vi "create checkpoint file name.vi"(8 "error in (no error)":errorcluster, 10 "name or relative path":string, 11 "Autofocus in":refnum<class "Autofocus.lvclass">) -> (0 "error out":errorcluster, 1 "checkpoint file name":path, 3 "Autofocus out":refnum<class "Autofocus.lvclass">)   [LabVIEW 2012, in "Autofocus.lvclass"]
uses:
  Autofocus.lvclass
  Autofocus.lvclass/Autofocus.ctl
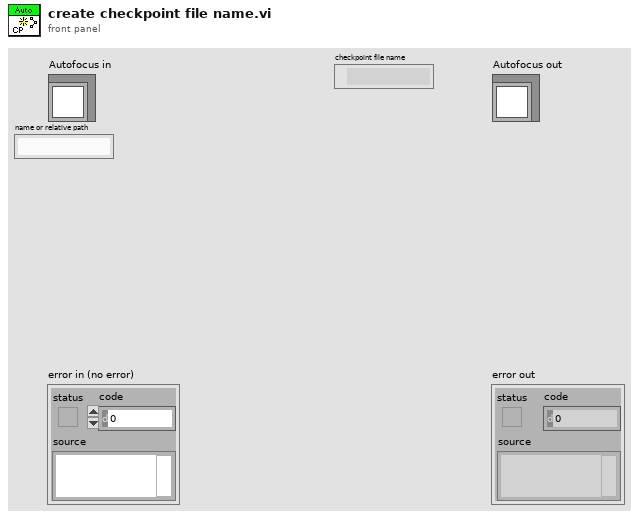
[diagram p1: front panel]
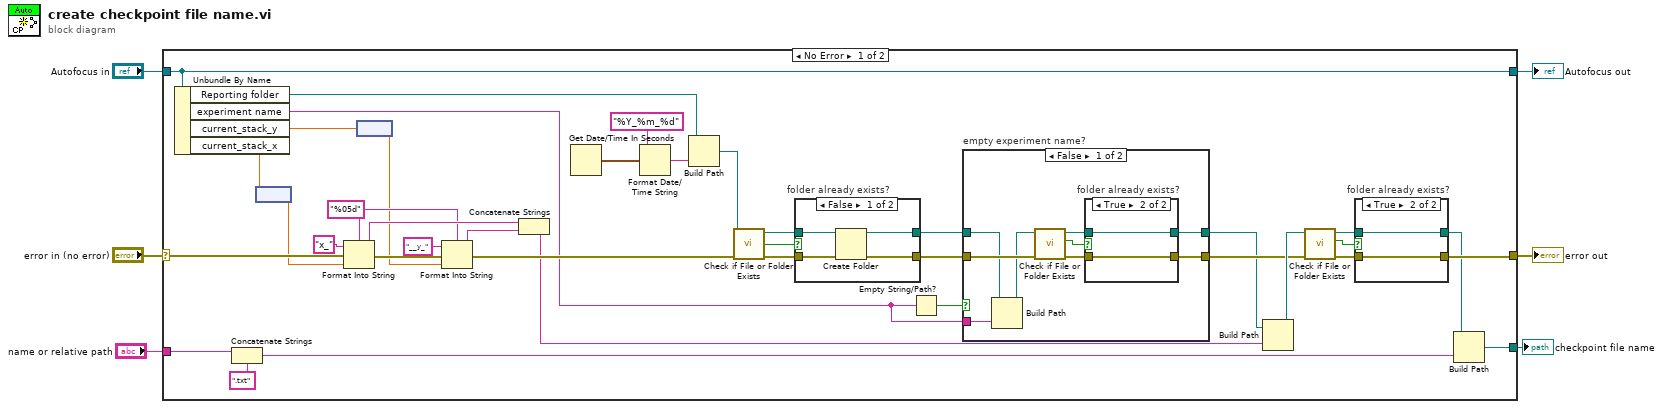
[diagram p0: block diagram]
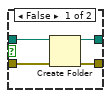
[diagram p2: hidden frame]
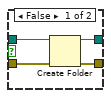
[diagram p4: hidden frame]
diagram:
  n1 = case shown="No Error" "error in (no error)" {
    selector: "error in (no error)" -> [w35 w75]
    tunnel: [w23 w75] -> w5
    tunnel: [w44 w74] -> w3
    tunnel: "Autofocus in" -> [w44 w74]
    tunnel: [w24 _] -> w2
    tunnel: "name or relative path" -> [w21 _]
    frame No Error {
      w41 = "%05d" ("format string")
      n2 = Unbundle By Name(w44) -> ("Reporting folder"=w31:path, "experiment name"=w8:string, "current_stack_y"=w36:dbl[unit], "current_stack_x"=w37:dbl[unit])
      n3 = Concatenate Strings(w21, ".txt" ("element")) -> (w19:string)
      n4 = node(w37) -> (w14:dbl)
      n5 = Format Into String(format string=w41, initial string="x_", error in=w35, w14) -> (resulting string=w42:string, error out=w38:errorcluster)
      n6 = node(w36) -> (w13:dbl)
      n7 = Format Into String(format string=w41, initial string="__y_", error in=w38, w13) -> (resulting string=w43:string, error out=w27:errorcluster)
      n8 = Concatenate Strings(w42, w43) -> (w25:string)
      n9 = Get Date/Time In Seconds() -> (seconds since 1Jan1904=w32:timestamp)
      n10 = Format Date/Time String(time format string (%c)="%Y_%m_%d", seconds (now)=w32) -> (date/time string=w34:string)  [unwired: 1 in]
      n11 = Build Path(base path=w31, name or relative path=w34) -> (appended path=w26:path)
      n12 = call <vilib>:"Check if File or Folder Exists.vi"("error in (no error)"=w27, "path"=w26) -> ("error out"=w29:errorcluster, "file or folder exists?"=w28:bool, "dup path"=w30:path)  [unwired: 7 in]
      n13 = case "folder already exists?" shown="False" w28 {
        tunnel: [w69 w73] -> w11
        tunnel: w29 -> [w71 w73]
        tunnel: w30 -> [w70 w72]
        tunnel: [w68 w72] -> w10
        frame False {
          n14 = Create Folder(path (use dialog)=w70, error in=w71) -> (created path=w68:path, error out=w69:errorcluster)  [unwired: 1 in, 1 out]
        }
        frame True {
        }
      }
      n15 = Empty String/Path?(string/path=w8) -> (empty?=w7:bool)
      n16 = case "empty experiment name?" shown="False" w7 {
        tunnel: [w50 w60] -> w12
        tunnel: w11 -> [w49 w60]
        tunnel: w10 -> [w48 w61]
        tunnel: [w46 w61] -> w9
        tunnel: w8 -> [w45 _]
        frame False {
          n17 = Build Path(base path=w48, name or relative path=w45) -> (appended path=w47:path)
          n18 = call <vilib>:"Check if File or Folder Exists.vi"("error in (no error)"=w49, "path"=w47) -> ("error out"=w53:errorcluster, "file or folder exists?"=w51:bool, "dup path"=w52:path)  [unwired: 7 in]
          n19 = case "folder already exists?" shown="True" w51 {
            tunnel: [w55 w59] -> w50
            tunnel: w53 -> [w57 w59]
            tunnel: w52 -> [w56 w58]
            tunnel: [w54 w58] -> w46
            frame False {
              n20 = Create Folder(path (use dialog)=w56, error in=w57) -> (created path=w54:path, error out=w55:errorcluster)  [unwired: 1 in, 1 out]
            }
            frame True {
            }
          }
        }
        frame True {
        }
      }
      n21 = Build Path(base path=w9, name or relative path=w25) -> (appended path=w17:path)
      n22 = call <vilib>:"Check if File or Folder Exists.vi"("error in (no error)"=w12, "path"=w17) -> ("error out"=w18:errorcluster, "file or folder exists?"=w15:bool, "dup path"=w16:path)  [unwired: 7 in]
      n23 = case "folder already exists?" shown="True" w15 {
        tunnel: [w63 w67] -> w23
        tunnel: w18 -> [w65 w67]
        tunnel: w16 -> [w64 w66]
        tunnel: [w62 w66] -> w22
        frame False {
          n24 = Create Folder(path (use dialog)=w64, error in=w65) -> (created path=w62:path, error out=w63:errorcluster)  [unwired: 1 in, 1 out]
        }
        frame True {
        }
      }
      n25 = Build Path(base path=w22, name or relative path=w19) -> (appended path=w24:path)
    }
    frame Error {
    }
  }
  "error out" <- w5
  "Autofocus out" <- w3
  "checkpoint file name" <- w2
